vi "RT Connect Streams.vi"(8 "error in (no error)":errorcluster) -> (0 "error out":errorcluster, 2 "reader endpoint":refnum<k21>, 3 "writer endpoint":refnum<k21>)   [LabVIEW 2021]
uses:
  Global Variables/RT GV.vi
  Global Variables/Network Globals.vi
panel:
  in  "timeout in ms (-1)":i32=1000
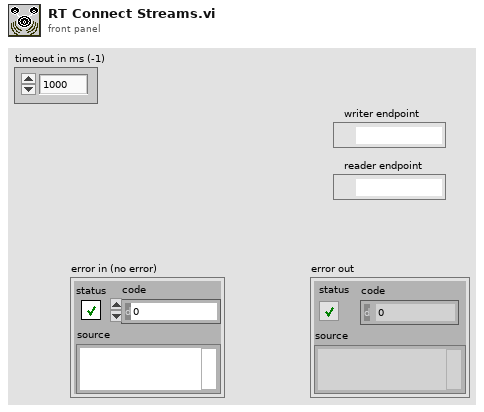
[diagram p1: front panel]
types:
  T1 = cluster{"Message":string, "Message Data":variant}
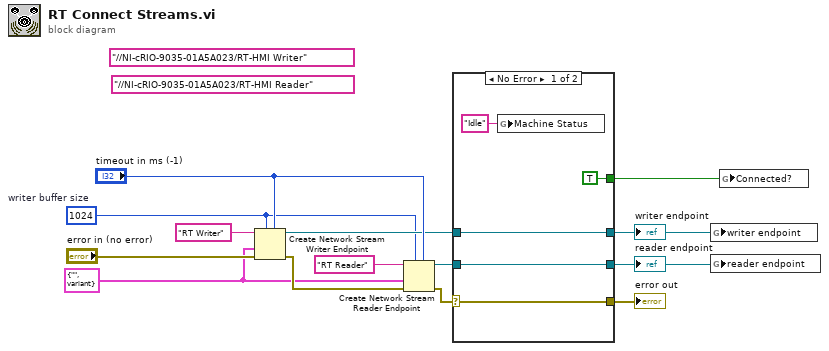
[diagram p0: block diagram]
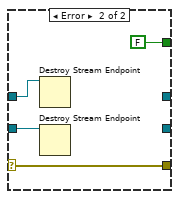
[diagram p2: hidden frame]
diagram:
  (unwired) "//NI-cRIO-9035-01A5A023/RT-HMI Writer" ("writer name")
  (unwired) "//NI-cRIO-9035-01A5A023/RT-HMI Reader" ("writer name")
  w4 = 1024  # writer buffer size
  w5 = T1 {"Message"="", "Message Data"=variant} ("Message Cluster")
  n1 = Create Network Stream Writer Endpoint(5:"timeout in ms (-1)", 7:w4, 8:"error in (no error)", 9:w5, 11:"RT Writer" ("writer name")) -> (0:w10:errorcluster, 3:w7:refnum<k21>)  [unwired: 2 in]
  n2 = Create Network Stream Reader Endpoint(5:"timeout in ms (-1)", 7:w4, 8:w10, 9:w5, 11:"RT Reader" ("reader name")) -> (0:w9:errorcluster, 3:w6:refnum<k21>)  [unwired: 2 in]
  n3 = case shown="No Error" w9 {
    selector: w9 -> [w19 w21]
    tunnel: [w19 w21] -> w8
    tunnel: w7 -> [w18 w23]
    tunnel: [w18 _] -> w3
    tunnel: w6 -> [w17 w22]
    tunnel: [w17 _] -> w2
    tunnel: [TRUE FALSE] -> w1
    frame No Error {
      n4 = global write "RT GV.vi" "Machine Status"("Idle" ("Machine Status")) -> ()
    }
    frame Error {
      n5 = Destroy Stream Endpoint(11:w23) -> ()  [unwired: 1 in, 1 out]
      n6 = Destroy Stream Endpoint(11:w22) -> ()  [unwired: 1 in, 1 out]
    }
  }
  "error out" <- w8
  "reader endpoint" <- w2
  "writer endpoint" <- w3
  n7 = global write "Network Globals.vi" "writer endpoint"(w3) -> ()
  n8 = global write "Network Globals.vi" "reader endpoint"(w2) -> ()
  n9 = global write "Network Globals.vi" "Connected?"(w1) -> ()
